vi "LINAKGetStatus.vi"(8 "Error In":errorcluster, 11 "MB_Master_TCP in":refnum<class "MB_Master_TCP.lvclass">) -> (0 "Error Out":errorcluster, 2 "StatusCluster":T1, 3 "MB_Master_TCP out":refnum<class "MB_Master_TCP.lvclass">)   [LabVIEW 2021]
uses:
  <vilib>/Plasmionique/MB Master/MB_Master_TCP/MB_Master_TCP.lvclass
  Applications/National Instruments/LabVIEW 2021 64-bit/vi.lib/Plasmionique/MB Master/MB_Master/MB_Master.lvclass
  LINAKStatusCluster.ctl
  <vilib>/Plasmionique/MB Master/MB Master.lvlib
panel:
  out "GoodToGo":bool
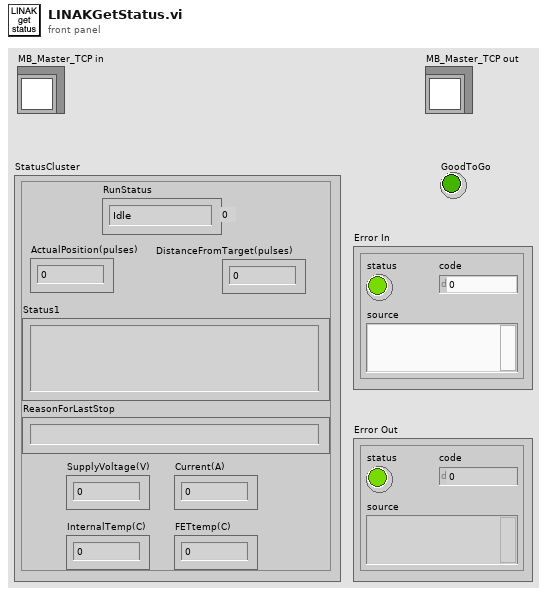
[diagram p1: front panel]
types:
  T1 = typedef "LINAKStatusCluster.ctl" = cluster{"RunStatus":enum16{"Idle", "RunningOut", "RunningIn", "WaitingToRun", "InitOut", "InitIn"}, "ActualPosition(pulses)":u16, "DistanceFromTarget(pulses)":u16, "Status1":string, "ReasonForLastStop":string, "SupplyVoltage(V)":dbl, "Current(A)":dbl, "InternalTemp(C)":i16, "FETtemp(C)":i16}
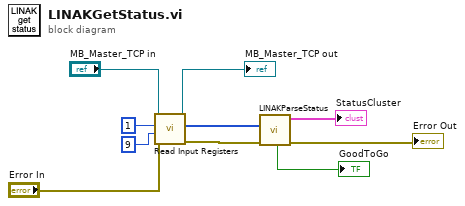
[diagram p0: block diagram]
diagram:
  n1 = call <vilib>:"Read Input Registers.vi"("error in (no error)"="Error In", "quantity"=u16 9, "starting address"=u16 1, "MB session in"="MB_Master_TCP in") -> ("error out"=w3:errorcluster, "Registers"=w6:u16[], "MB session out"=→"MB_Master_TCP out":refnum<class "MB_Master_TCP.lvclass">)  [unwired: 5 in]
  n2 = call "LINAKParseStatus.vi"("Error In"=w3, "Registers"=w6) -> ("Error Out"=→"Error Out":errorcluster, "StatusCluster"=→"StatusCluster":T1, "GoodToGo"=→"GoodToGo":bool)  [unwired: 7 in]
